vi "Subvi AO trigger 20180613.vi"(10 "Ext trigger":bool) -> (2 "Boolean":bool)   [LabVIEW 2017]
uses:
  <vilib>/Platform/TimedLoop/XDataNode/timing_clust.ctl
  <vilib>/Platform/TimedLoop/XDataNode/nitl_modes.ctl
  <vilib>/Platform/TimedLoop/XDataNode/wakeup.ctl
  <vilib>/rvi/Emulation/niFpgaSctlEmulationGetInTimedLoop.vi
  <vilib>/rvi/Emulation/niFpgaEmulationReportErrorSimple.vi
  <vilib>/rvi/Emulation/niFpgaGetClockAttributes.vi
  <vilib>/rvi/Emulation/niFpgaCriticalErrorInLSC.vi
  Detector/GV frameclock.vi
  Detector/GV frame counter.vi
  <vilib>/Platform/TimedLoop/XDataNode/XDataNode.xnode
  <vilib>/Platform/TimedLoop/XDataNode/XDNodeRunTimeDep.lvlib
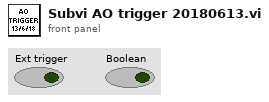
[diagram p1: front panel]
types:
  T1 = typedef "XDNodeRunTimeDep.lvlib/timing_clust.ctl" = cluster{"Expected End [f-1]":u64, "Actual End [f-1]":u64, "Finished Late? [f-1]":bool, "Expected End [i-1]":u64, "Actual End [i-1]":u64, "Finished Late? [i-1]":bool, "Expected Start [i]":u64, "Actual Start [i]":u64, "Expected Start [f]":u64, "Actual Start [f]":u64, "Source Name":string, "Structure Name":string, "Period":i64, "Deadline":i64, "Offset":i64, "Start":i64, "Priority":i32, "Timeout":i32, "Mode":T2, "Wakeup Reason":T3, "Error":errorcluster, "Source Type":string, "Secondary Source Type":string, "Global End Time":u64, "Global Start Time":u64, "Frame Duration":u64, "Iteration Duration":u64, "Assigned CPU":i32, "I/O Scan Engine Mode":u32}
  T2 = typedef "XDNodeRunTimeDep.lvlib/nitl_modes.ctl" = enum32{"No Change", "Process missed periods, maintain original phase", "Discard missed periods, maintain original phase", "Process missed periods, ignore original phase", "Discard missed periods, ignore original phase"}
  T3 = typedef "XDNodeRunTimeDep.lvlib/wakeup.ctl" = enum32{"Normal", "Aborted", "Asynchronous wakeup", "Timing source error", "Timed loop error", "Timeout"}
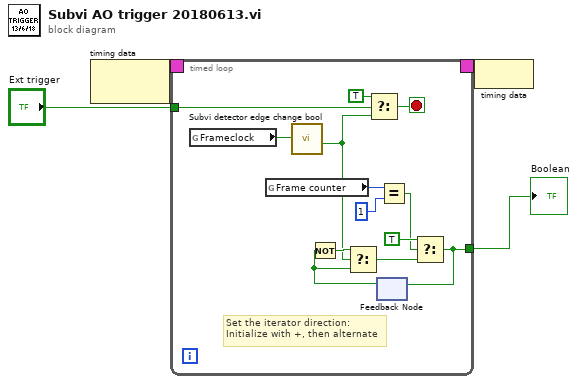
[diagram p0: block diagram]
diagram:
  n1 = node-c288() -> (w4:T1)  [unwired: 1 in]
  n2 = timed-loop {
    timing: w4 -> [_]
    timing-out: [_] -> w3
    tunnel: [w7] -> w1
    tunnel: "Ext trigger" -> [w5]
    stop <- w17 stop-if-true
    # "Set the iterator direction:\nInitialize with +, then alternate"
    n3 = global read "GV frameclock.vi" "Frameclock"() -> (w15:bool)
    n4 = global read "GV frame counter.vi" "Frame counter"() -> (w11:u8)
    n5 = call "Subvi detector edge change bool.vi"("Input"=w15) -> ("Output"=w12:bool)  [unwired: 8 in]
    n6 = Select(t=TRUE, s=w5, f=w12) -> (s? t:f=w17:bool)
    n7 = feedback #1() -> (w6:bool)  [unwired: 1 in]
    n8 = Not(x=w6) -> (.not. x?=w13:bool)
    n9 = Select(t=w13, s=w12, f=w6) -> (s? t:f=w8:bool)
    n10 = Equal?(x=w11, y=u8 1) -> (x = y?=w9:bool)
    n11 = Select(t=TRUE, s=w9, f=w8) -> (s? t:f=w7:bool)
    n12 = feedback-in #1(w7) -> ()
  }
  "Boolean" <- w1
  n13 = node-c288(w3) -> ()
